vi "GetText.vi"(8 "error in":errorcluster, 11 "node in":refnum<class "Bus.lvclass">) -> (0 "error out":errorcluster, 1 "additional text":string, 2 "text":string, 3 "node out":refnum<class "Bus.lvclass">, 4 "glyph":string)   [LabVIEW 2014, in "Bus.lvclass"]
doc: "Returns the text representation of the node used for the tree control."
uses:
  Bus.lvclass
  Bus.lvclass/Bus.ctl
  <vilib>/NI/Configuration Framework/serializable configuration/NISE_CEF_serializable configuration.lvclass
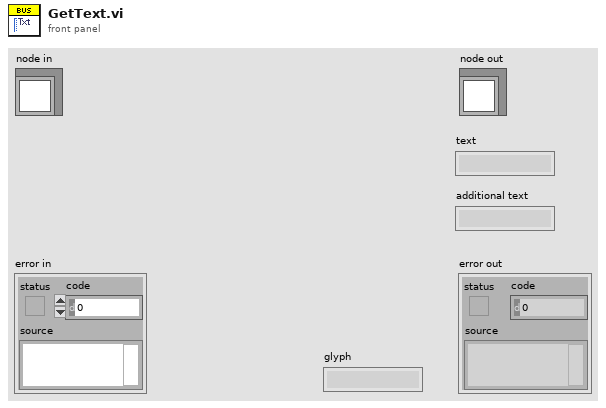
[diagram p1: front panel]
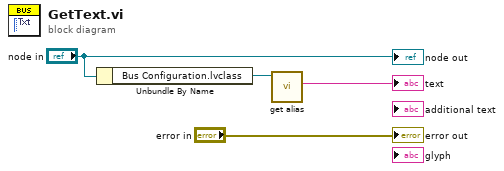
[diagram p0: block diagram]
diagram:
  n1 = Unbundle By Name("node in") -> ("Bus Configuration.lvclass"=w4:refnum<class "Bus Configuration.lvclass">)
  n2 = call <vilib>:"get alias.vi"("configuration in"=w4) -> ("alias"=→"text":string)  [unwired: 8 in, 2 out]
  "error out" <- "error in"
  "node out" <- "node in"
